vi "Init Hardware.vi"(8 "error in (no error)":errorcluster, 11 "Keithley 622x Driver in":refnum<class "Keithley 622x2182 Driver.lvclass">) -> (0 "error out":errorcluster, 3 "Keithley 622x Driver out":refnum<class "Keithley 622x2182 Driver.lvclass">)   [LabVIEW 2021, in "Keithley 622x2182 Driver.lvclass"]
uses:
  Keithley 622x2182 Driver.lvclass
  C:/GitHub/NHMFL_Core/Libraries/Instruments/VISA Instrument/VISA Instrument.lvclass
  C:/GitHub/NHMFL_Core/Libraries/Instruments/Instrument Driver/Instrument Driver.lvclass
  VISA Instrument/VISA Instrument.lvclass/VISA Instrument.ctl
  Keithley 622x2182 Driver.lvclass/Keithley 622x2182 Driver.ctl
  Instrument Driver/Instrument Driver.lvclass/Instrument Driver.ctl
  VISA Instrument/Read VISA resource.vi
  VISA Instrument/Write VISA resource.vi
  Instrument Driver/Write Channel names.vi
  Instrument Driver/Write Channel units.vi
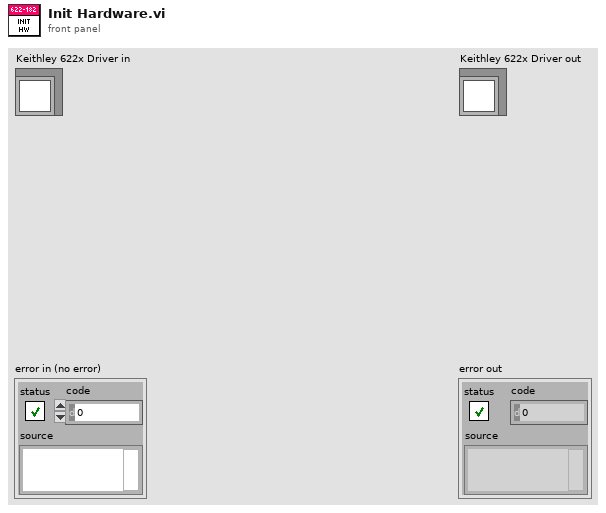
[diagram p1: front panel]
types:
  T1 = typedef "Stepper Config.ctl" = cluster{"Start":dbl, "End":dbl, "Step":dbl, "Delta":dbl, "Scan shape":enum16{"Sawtooth", "Triangular"}, "Append measurements":string[], "Pulse width":dbl, "Pulse interval":dbl, "Scan mode":enum16{"Delta", "Diff. conductance", "Pulse delta sweep"}}
  T2 = enum16{"Delta", "Diff. conductance", "Pulse delta sweep"}
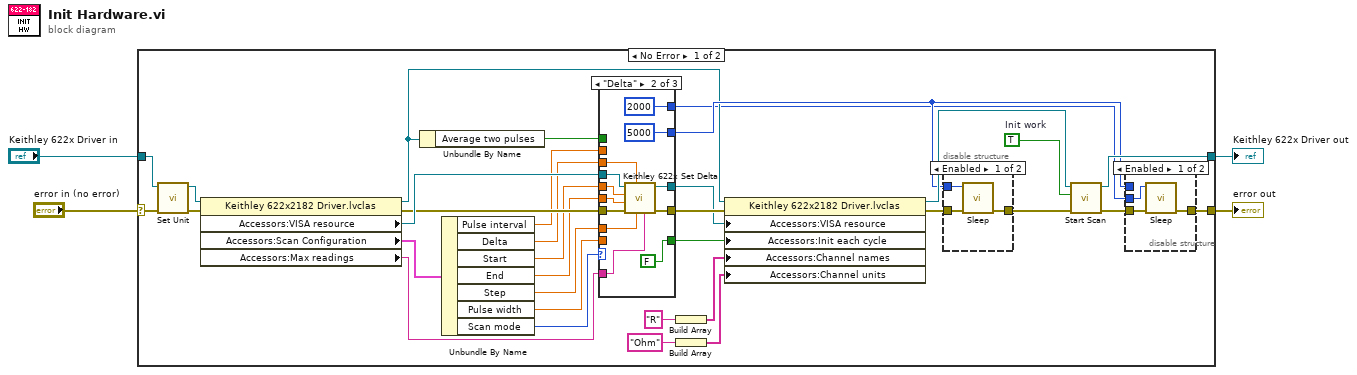
[diagram p0: block diagram]
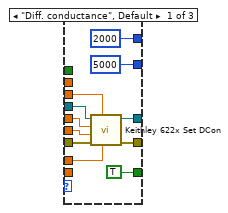
[diagram p3: hidden frame]
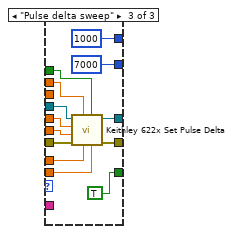
[diagram p4: hidden frame]
diagram:
  n1 = case shown="No Error" "error in (no error)" {
    selector: "error in (no error)" -> [w6 w83]
    tunnel: "Keithley 622x Driver in" -> [w8 w82]
    tunnel: [w35 w82] -> w3
    tunnel: [w23 w83] -> w2
    frame No Error {
      w12 = TRUE  # Init work
      n2 = call-dynamic "Set Unit.vi"("error in (no error)"=w6, "Keithley 622x2182 Driver in"=w8) -> ("error out"=w5:errorcluster, "Keithley 622x2182 Driver out"=w7:refnum<class "Keithley 622x2182 Driver.lvclass">)  [unwired: 8 in]
      n3 = property class="Keithley 622x2182 Driver.lvclas"(reference=w7, error in=w5) -> (reference out=w18:refnum<class "Keithley 622x2182 Driver.lvclass">, error out=w33:errorcluster, "Accessors:VISA resource"=w34:refnum<visa-resource-name>, "Accessors:Scan Configuration"=w37:T1, "Accessors:Max readings"=w11:string)
      n4 = Unbundle By Name(w18) -> ("Average two pulses"=w17:bool)
      n5 = Unbundle By Name(w37) -> ("Pulse interval"=w24:dbl, "Delta"=w28:dbl, "Start"=w30:dbl, "End"=w29:dbl, "Step"=w27:dbl, "Pulse width"=w25:dbl, "Scan mode"=w26:T2)
      n6 = case shown="\"Delta\"" w26 {
        tunnel: w34 -> [w52 w64 w74]
        tunnel: w33 -> [w51 w63 w77]
        tunnel: [w50 w62 w76] -> w32
        tunnel: [w49 w61 w75] -> w31
        tunnel: w30 -> [w48 w60 w71]
        tunnel: w29 -> [w47 w59 w70]
        tunnel: w28 -> [w46 w58 _]
        tunnel: w27 -> [w45 w57 w69]
        tunnel: w24 -> [_ _ w73]
        tunnel: w25 -> [_ _ w72]
        tunnel: [u32 5000 ("milliseconds to wait") u32 5000 ("milliseconds to wait") u32 7000 ("milliseconds to wait")] -> w19
        tunnel: w17 -> [_ _ w67]
        tunnel: [u32 2000 ("milliseconds to wait") u32 2000 ("milliseconds to wait") u32 1000 ("milliseconds to wait")] -> w13
        tunnel: w11 -> [_ w54 _]
        tunnel: [TRUE ("Init each cycle") FALSE ("Init each cycle") TRUE ("Init each cycle")] -> w9
        frame "Diff. conductance", Default {
          n7 = call "Keithley 622x Set DCon.vi"("Step"=w45, "Delta"=w46, "error in"=w51, "End"=w47, "Start"=w48, "VISA resource name"=w52) -> ("error out"=w50:errorcluster, "VISA resource name out"=w49:refnum<visa-resource-name>)  [unwired: 4 in]
        }
        frame "Delta" {
          n8 = call "Keithley 622x Set Delta.vi"("Max readings"=w54, "Step"=w57, "Delta"=w58, "error in"=w63, "End"=w59, "Start"=w60, "VISA resource name"=w64) -> ("error out"=w62:errorcluster, "VISA resource name out"=w61:refnum<visa-resource-name>)  [unwired: 3 in]
        }
        frame "Pulse delta sweep" {
          n9 = call "Keithley 622x Set Pulse Delta.vi"("Width"=w72, "Average two pulses"=w67, "Step"=w69, "Delay"=w73, "error in"=w77, "End"=w70, "Start"=w71, "VISA resource name"=w74) -> ("error out"=w76:errorcluster, "VISA resource name out"=w75:refnum<visa-resource-name>)  [unwired: 2 in]
        }
      }
      n10 = Build Array("R" ("String")) -> (w10:string[])
      n11 = Build Array("Ohm" ("String")) -> (w15:string[])
      n12 = property class="Keithley 622x2182 Driver.lvclas"(reference=w18, error in=w32, "Accessors:VISA resource"=w31, "Accessors:Init each cycle"=w9, "Accessors:Channel names"=w10, "Accessors:Channel units"=w15) -> (reference out=w36:refnum<class "Keithley 622x2182 Driver.lvclass">, error out=w21:errorcluster)
      n13 = disable-structure shown="Enabled" {
        disable-tunnel: [w40 w41] -> w20
        disable-tunnel: w19 -> [w39 _]
        disable-tunnel: w21 -> [w38 w41]
        frame Enabled {
          n14 = call "Sleep.vi"("error in"=w38, "milliseconds to wait"=w39) -> ("error out"=w40:errorcluster)  [unwired: 9 in]
        }
        frame Disabled {
        }
      }
      n15 = call-dynamic "Start Scan.vi"("error in (no error)"=w20, "Init work"=w12, "Keithley 622x2182 Driver in"=w36) -> ("error out"=w22:errorcluster, "Keithley 622x2182 Driver out"=w35:refnum<class "Keithley 622x2182 Driver.lvclass">)  [unwired: 7 in]
      n16 = disable-structure shown="Enabled" {
        disable-tunnel: [w80 w81] -> w23
        disable-tunnel: w22 -> [w79 w81]
        disable-tunnel: w19 -> [_ _]
        disable-tunnel: w13 -> [w78 _]
        frame Enabled {
          n17 = call "Sleep.vi"("error in"=w79, "milliseconds to wait"=w78) -> ("error out"=w80:errorcluster)  [unwired: 9 in]
        }
        frame Disabled {
        }
      }
    }
    frame Error {
    }
  }
  "error out" <- w2
  "Keithley 622x Driver out" <- w3
